vi "Spectrograph_getEvent_disperserReportedPosition.vi"(8 "error in (no error)":errorcluster, 11 "logevent_disperserReportedPosition_Ctl":T1) -> (0 "error out":errorcluster, 2 "function return":i32, 3 "logevent_disperserReportedPosition_Ctl out":T1)   [LabVIEW 2016, in "SALLV_Spectrograph.lvlib"]
doc: "int Spectrograph_shm_getEvent_disperserReportedPositionLV(Spectrograph_logevent_disperserReportedPositionLV *logevent_disperserReportedPosition_Ctl );"
uses:
  SALLV_Spectrograph.lvlib
  DataTypes/logevent_disperserReportedPosition.ctl
  SALLV_Spectrograph.so
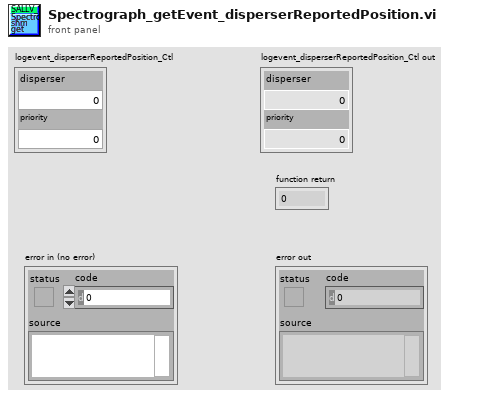
[diagram p1: front panel]
types:
  T1 = typedef "SALLV_Spectrograph.lvlib/logevent_disperserReportedPosition.ctl" = cluster{"disperser":i32, "priority":i32}
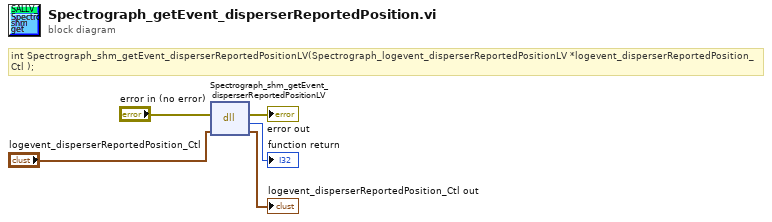
[diagram p0: block diagram]
diagram:
  # "int Spectrograph_shm_getEvent_disperserReportedPositionLV(Spectrograph_logevent_disperserReportedPositionLV *logevent_disperserReportedPosition_Ctl );"
  n1 = dll-call lib="home/harini/TCS/SALLV_Spectrograph/SALLV_Spectrograph.*" fn="Spectrograph_shm_getEvent_disperserReportedPositionLV"(error in="error in (no error)", "logevent_disperserReportedPosition_Ctl"="logevent_disperserReportedPosition_Ctl") -> (error out=→"error out":errorcluster, →"function return":i32, "logevent_disperserReportedPosition_Ctl"=→"logevent_disperserReportedPosition_Ctl out":T1)  [unwired: 2 in, 1 out]
